vi "UI-message-handler.vi"(8 "error in (no error)":errorcluster, 9 "Additional text":string, 10 "Message":T2, 11 "Language":T1) -> (0 "error out":errorcluster)   [LabVIEW 2013, in "Client.lvlib" / "Client.lvclass"]
doc: "Displays a predefined message to the user.\nThe default display type is a one-button dialog.\n\nThe possible types of UI messages are specified by the 'UI-messages' type definition."
uses:
  Client.lvclass
  UI-messages.ctl
  Languages.ctl
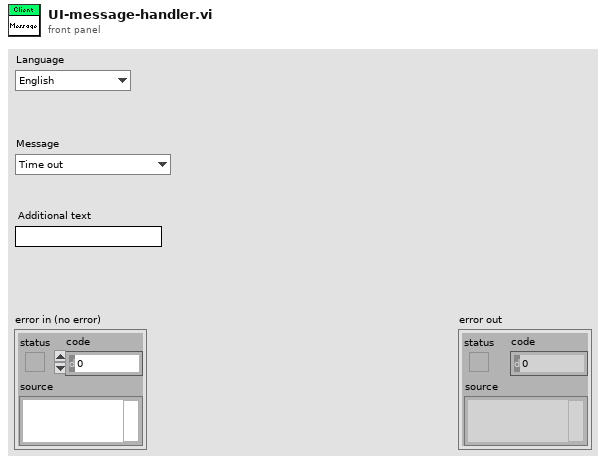
[diagram p1: front panel]
types:
  T1 = typedef "Client.lvlib/Client.lvclass/Languages.ctl" = enum16{"English"}
  T2 = typedef "Client.lvlib/Client.lvclass/UI-messages.ctl" = enum16{"Time out", "User cancel", "Module cancel"}
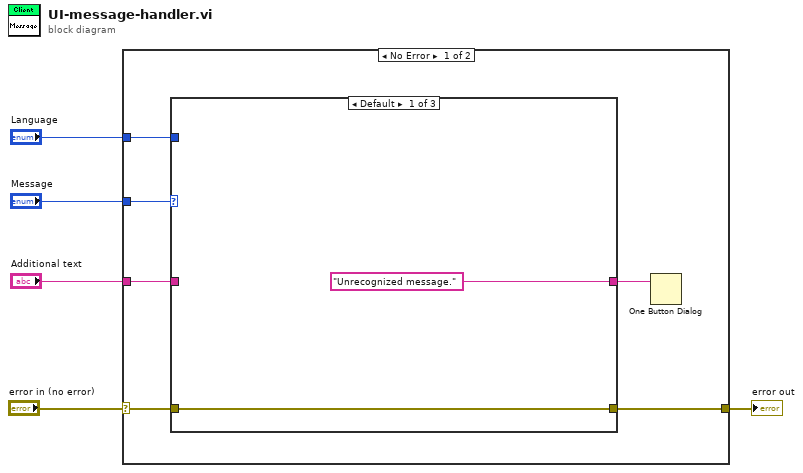
[diagram p0: block diagram]
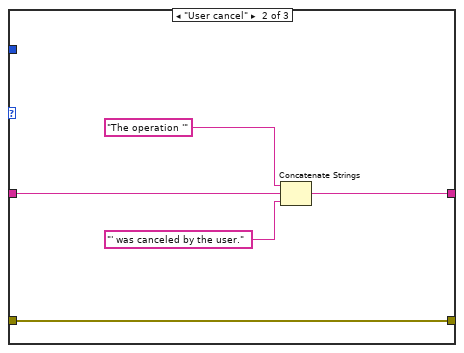
[diagram p2: hidden frame]
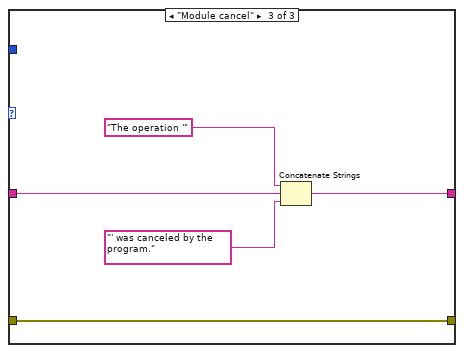
[diagram p3: hidden frame]
diagram:
  n1 = case shown="No Error" "error in (no error)" {
    selector: "error in (no error)" -> [w11 w24]
    tunnel: [w8 w24] -> w4
    tunnel: "Message" -> [w10 _]
    tunnel: "Additional text" -> [w9 _]
    tunnel: "Language" -> [w6 _]
    frame No Error {
      n2 = case shown="Default" w10 {
        tunnel: w11 -> [w13 w18 w23]
        tunnel: w9 -> [_ w17 w22]
        tunnel: [w13 w18 w23] -> w8
        tunnel: ["Unrecognized message." w14 w19] -> w7
        tunnel: w6 -> [_ _ _]
        frame Default {
        }
        frame "User cancel" {
          n3 = Concatenate Strings("The operation '", w17, "' was canceled by the user.") -> (w14:string)
        }
        frame "Module cancel" {
          n4 = Concatenate Strings("The operation '", w22, "' was canceled by the program.") -> (w19:string)
        }
      }
      n5 = One Button Dialog(message=w7) -> ()  [unwired: 1 in, 1 out]
    }
    frame Error {
    }
  }
  "error out" <- w4
